vi "Protocol Read.vi"(8 "error in (no error)":errorcluster, 9 "timeout":i32=10000, 10 "bytes to read":i32, 11 "protocol layer in":refnum<class "TCP Slave.lvclass">) -> (0 "error out":errorcluster, 1 "timed out?":bool, 2 "data":u8[](array[numeric]), 3 "protocol layer out":refnum<class "TCP Slave.lvclass">)   [LabVIEW 2018, in "SubVIs.lvlib" / "TCP Slave.lvclass"]
doc: "Reads from the established TCP connection stored in the class."
uses:
  TCP Slave.lvclass
  TCP Slave.lvclass/TCP Slave.ctl
  TCP Shared Components.lvlib
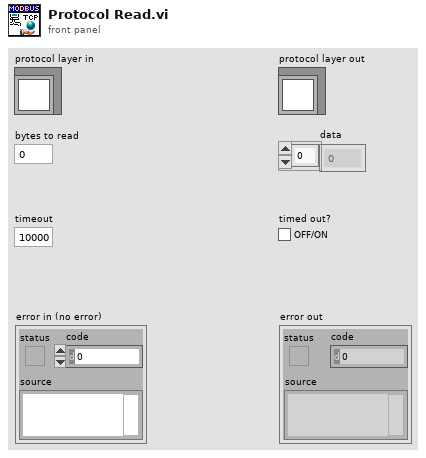
[diagram p1: front panel]
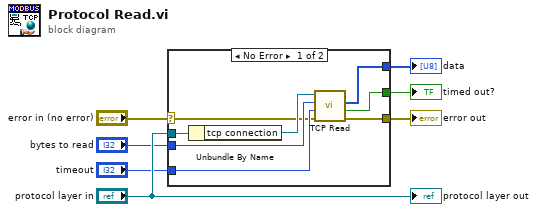
[diagram p0: block diagram]
diagram:
  n1 = case shown="No Error" "error in (no error)" {
    selector: "error in (no error)" -> [w8 w16]
    tunnel: "protocol layer in" -> [w15 _]
    tunnel: "bytes to read" -> [w13 _]
    tunnel: "timeout" -> [w12 _]
    tunnel: [w11 w16] -> w4
    tunnel: [w10 _] -> w3
    tunnel: [w9 _] -> w2
    frame No Error {
      n2 = Unbundle By Name(w15) -> ("tcp connection"=w14:refnum<k5>)
      n3 = call "TCP Read.vi"("error in (no error)"=w8, "timeout"=w12, "bytes to read"=w13, "connection ID"=w14) -> ("error out"=w11:errorcluster, "timed out?"=w10:bool, "data"=w9:u8[])  [unwired: 5 in]
    }
    frame Error {
    }
  }
  "error out" <- w4
  "data" <- w2
  "timed out?" <- w3
  "protocol layer out" <- "protocol layer in"
